vi "subPopulateRulesParserSelector.vi"(8 "error in (no error)":errorcluster, 10 "Selection":string, 11 "UIManager in":refnum<class "UIManager.lvclass">) -> (0 "error out":errorcluster, 1 "Display name":string, 2 "Rule parser names":string[](array[string]), 3 "UIManager out":refnum<class "UIManager.lvclass">)   [LabVIEW 2020, in "UserInterface.lvlib" / "UIManager.lvclass"]
uses:
  UIManager.lvclass
  UIManager.lvclass/UIManager.ctl
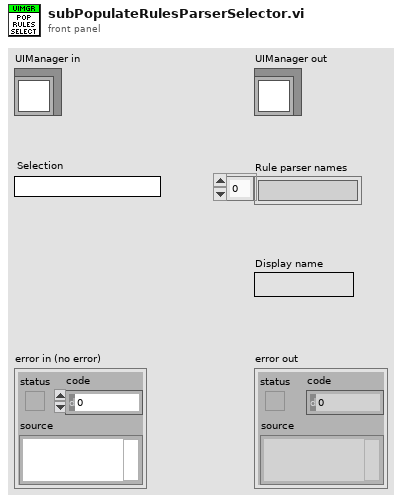
[diagram p1: front panel]
types:
  T1 = map{string, refnum<class "IRuleFileParser.lvclass">}
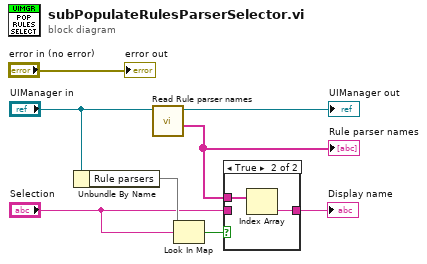
[diagram p0: block diagram]
diagram:
  n1 = Unbundle By Name("UIManager in") -> ("Rule parsers"=w4:T1)
  n2 = call-dynamic "Read Rule parser names.vi"("UIManager in"="UIManager in") -> ("Rule parser names"=w7:string[], "UIManager out"=→"UIManager out":refnum<class "UIManager.lvclass">)  [unwired: 9 in]
  "Rule parser names" <- w7
  n3 = Look In Map(map=w4, key="Selection") -> (key not found?=w3:bool)  [unwired: 1 in, 1 out]
  n4 = case shown="True" w3 {
    tunnel: w7 -> [_ w11]
    tunnel: [w9 w10] -> w1
    tunnel: "Selection" -> [w9 _]
    frame False {
    }
    frame True {
      n5 = Index Array(array=w11) -> (element=w10:string)  [unwired: 1 in]
    }
  }
  "Display name" <- w1
  "error out" <- "error in (no error)"
